vi "SaccadeAnalyser - Replace Rotation Vector Data Channels With Angles.vi"(10 "Sample Rate (Hz)":dbl=500.0, 11 "Data Channels (in)":dbl[][](array[numeric])) -> (3 "Data Channels (out)":dbl[][](array[numeric]))   [LabVIEW 2016]
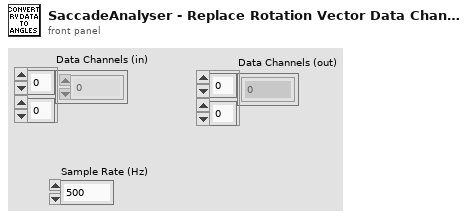
[diagram p1: front panel]
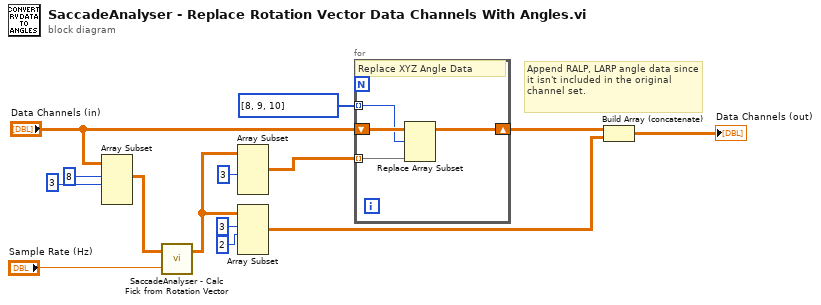
[diagram p0: block diagram]
diagram:
  # "Append RALP, LARP angle data since it isn't included in the original channel set."
  n1 = Array Subset(array="Data Channels (in)", index (row)=8 ("index"), length (row)=3 ("length")) -> (w11:dbl[][])  [unwired: 2 in]
  n2 = call "SaccadeAnalyser - Calc Fick from Rotation Vector.vi"("Sample Rate (Hz)"="Sample Rate (Hz)", "Rotation Vectors (XYZ)"=w11) -> ("Angles Roll, Pitch, Yaw, RALP, LARP (deg)"=w6:dbl[][])  [unwired: 1 out]
  n3 = Array Subset(array=w6, length (row)=3 ("length")) -> (w7:dbl[][])  [unwired: 3 in]
  n4 = Array Subset(array=w6, index (row)=3 ("index"), length (row)=2 ("length")) -> (w2:dbl[][])  [unwired: 2 in]
  n5 = for {
    shift-right: [w17] -> w3
    shift-left: "Data Channels (in)" -> [w18]
    tunnel: i32[] [8, 9, 10] -> [w16] mode=indexing
    tunnel: w7 -> [w15] mode=indexing
    # "Replace XYZ Angle Data"
    n6 = Replace Array Subset(array=w18, new element=w15, index (row)=w16) -> (w17:dbl[][])  [unwired: 1 in]
  }
  n7 = Build Array (concatenate)(w3, w2) -> (→"Data Channels (out)":dbl[][])
